vi "PJ1_GG.vi"() -> ()   [LabVIEW 2024]
uses:
  C:/Users/Windows 11/Downloads/Control 9.ctl
  <vilib>/Instr/_visa.llb/VISA Configure Serial Port (Instr).vi
  <vilib>/express/express analysis/Spectral/Block/exnSpectralBlock spectral measurements PSD poly.vi
  <vilib>/express/express analysis/Spectral/Block/exnSpectralBlock spectral measurements PSD DDT.vi
  <vilib>/express/express analysis/Spectral/XNode/ExpressSpectralMeasurementsBlockNode.xnode
panel:
  in  "Sample":i32
  in  "Rate":dbl
  out "EEG Str":string
  in  "Upper Cut-Off":dbl=40.0
  out "PSD":dynamicdata(graph)
  out "PSD MAX":dbl
  out "Index ที่มากที่สุด":i32
  out "max value":dbl
  out "B 18+1":dbl
  out "N 18+1":dbl
  in  "Aj 18+1":dbl
  out "B 18+1":dbl
  out "PSD 18+1":dbl
  out "B 18":dbl
  out "N 18":dbl
  in  "Aj 18":dbl
  out "B 18":dbl
  out "PSD 18":dbl
  out "B 18-1":dbl
  out "N 18-1":dbl
  in  "Aj 18-1":dbl
  out "B 18-1":dbl
  out "PSD 18-1":dbl
  out "9 Hz":dbl[](array[numeric])
  out "Max Index 9":i32
  out "PSD max 9":dbl
  out "PSD 9-1":dbl
  out "B 9-1":dbl
  in  "Aj 9-1":dbl
  out "N 9-1":dbl
  out "B 9-1":dbl
  out "PSD 9":dbl
  out "B 9":dbl
  in  "Aj 9":dbl
  out "N 9":dbl
  out "B 9":dbl
  out "PSD 9+1":dbl
  out "B 9+1":dbl
  in  "Aj 9+1":dbl
  out "N 9+1":dbl
  out "B 9+1":dbl
  out "8 Hz":dbl[](array[numeric])
  out "Max Index 8":i32
  out "PSD max 8":dbl
  out "B 16+1":dbl
  out "N 16+1":dbl
  in  "Aj  16+1":dbl
  out "B 16+1":dbl
  out "PSD  16+1":dbl
  out "B 16":dbl
  out "N  16":dbl
  in  "Aj  16":dbl
  out "B 16":dbl
  out "PSD  16":dbl
  out "B 16-1":dbl
  out "N  16-1":dbl
  in  "Aj   16-1":dbl
  out "B   16-1":dbl
  out "PSD 16-1":dbl
  out "B 8+1":dbl
  out "N 8+1":dbl
  in  "Aj  8+1":dbl
  out "B  8+1":dbl
  out "PSD 8+1":dbl
  out "B 8":dbl
  out "N  8":dbl
  in  "Aj  8":dbl
  out "B  8":dbl
  out "PSD 8":dbl
  out "B 8-1":dbl
  out "N  8-1":dbl
  in  "Aj  8-1":dbl
  out "B  8-1":dbl
  out "PSD 8-1":dbl
  out "PSD 14+1":dbl
  out "B 14+1":dbl
  in  "Aj 14+1":dbl
  out "N 14+1":dbl
  out "B 14+1":dbl
  out "PSD 14":dbl
  out "B 14":dbl
  in  "Aj 14":dbl
  out "N 14":dbl
  out "B 14":dbl
  out "PSD 14-1":dbl
  out "B 14-1":dbl
  in  "Aj 14-1":dbl
  out "N 14-1":dbl
  out "B 14-1":dbl
  out "PSD7+1":dbl
  out "B7+1":dbl
  in  "Aj7+1":dbl
  out "N7+1":dbl
  out "B7+1":dbl
  out "PSD 7":dbl
  out "B 7":dbl
  in  "Aj 7":dbl
  out "N7":dbl
  out "B7":dbl
  out "7 Hz":dbl[](array[numeric])
  out "Max Index 7":i32
  out "PSD max 7":dbl
  out "PSD 7-1":dbl
  out "B 7-1":dbl
  in  "Aj 7-1":dbl
  out "N7-1":dbl
  out "B7-1":dbl
  out "B12-1":dbl
  out "N12-1":dbl
  in  "Aj 12-1":dbl
  out "B 12-1":dbl
  out "PSD 12-1":dbl
  out "B12":dbl
  out "N12":dbl
  in  "Aj 12":dbl
  out "B12":dbl
  out "PSD 12":dbl
  out "B12+1":dbl
  out "N12+1":dbl
  in  "Aj 12+1":dbl
  out "B 12+1":dbl
  out "PSD 12+1":dbl
  out "B6+1":dbl
  out "N6+1":dbl
  in  "Aj 6+1":dbl
  out "B 6+1":dbl
  out "PSD 6+1":dbl
  out "B6":dbl
  out "N6":dbl
  in  "Aj 6":dbl
  out "B6":dbl
  out "PSD 6":dbl
  out "PSD 6-1":dbl
  out "6 Hz":dbl[](array[numeric])
  out "Max Index 6":i32
  out "PSD max 6":dbl
  out "B 6-1":dbl
  in  "Aj 6-1":dbl
  out "N6-1":dbl
  out "B6-1":dbl
  in  "Baseline":bool
  out "appended array":dbl[][](array[numeric])
  out "Filtered Signal":dynamicdata(graph)
  in  "Lower Cut-Off":dbl=1.0
  out "data":dbl[][](graph) caption="Raw Data"
  out "?":bool
  out "?":bool
  out "?":bool
  out "?":bool
  out "?":bool
  out "?":bool
  out "?":bool
  out "?":bool
  out "?":bool
  out "?":bool
  out "?":bool=TRUE
  out "?":bool=TRUE
  out "?":bool=TRUE
  out "?":bool=TRUE
  out "?":bool=TRUE
  out "?":bool=TRUE
  out "?":bool=TRUE
  out "?":bool=TRUE
  out "?":bool=TRUE
  out "?":bool=TRUE
  out "?":bool
  out "?":bool
  out "?":bool
  out "?":bool
  out "?":bool
  out "?":bool
  out "?":bool
  out "?":bool
  out "?":bool
  out "?":bool
  out "?":bool=TRUE
  out "?":bool=TRUE
  out "?":bool=TRUE
  out "?":bool=TRUE
  out "?":bool=TRUE
  out "?":bool=TRUE
  out "?":bool=TRUE
  out "?":bool=TRUE
  out "?":bool=TRUE
  out "?":bool=TRUE
  out "?":bool
  out "?":bool
  out "?":bool
  out "?":bool
  out "?":bool
  out "?":bool
  out "?":bool
  out "?":bool
  out "?":bool
  out "?":bool
  out "?":bool=TRUE
  out "?":bool=TRUE
  out "?":bool=TRUE
  out "?":bool=TRUE
  out "?":bool=TRUE
  out "?":bool=TRUE
  out "?":bool=TRUE
  out "?":bool=TRUE
  out "?":bool=TRUE
  out "?":bool=TRUE
  out "?":bool
  out "?":bool
  out "?":bool
  out "?":bool
  out "?":bool
  out "?":bool
  out "?":bool
  out "?":bool
  out "?":bool
  out "?":bool
  out "?":bool=TRUE
  out "?":bool=TRUE
  out "?":bool=TRUE
  out "?":bool=TRUE
  out "?":bool=TRUE
  out "?":bool=TRUE
  out "?":bool=TRUE
  out "?":bool=TRUE
  out "?":bool=TRUE
  out "?":bool=TRUE
  out "9 HZ":bool
  out "8 HZ":bool
  out "6 HZ":bool
  out "7 HZ":bool
  in  "Tab Control":enum32{"TAB 1", "TAB 2", "TAB 3", "TAB 4"}(tab)
  out "555":bool
  in  "MENU 4":bool
  in  "MENU 3":bool
  in  "MENU 2":bool
  in  "MENU":bool
  in  "start":bool
  in  "Text3":bool
  in  "Text2":bool
  in  "Backpage 2":T1
  out "String":string
  in  "Text1":bool
  in  "send":bool
  in  "Back":bool
  in  "1 3":bool
  in  "1 2":bool
  in  "1":bool
  out "String 2":string
  in  "SOS CALLING":bool
  in  "Blank Button 14":bool
  in  "LED":bool
  in  "Blank Button 12":bool
  in  "Back 4":bool
  in  "VISA resource name":refnum<visa-resource-name>
  # "Tel."
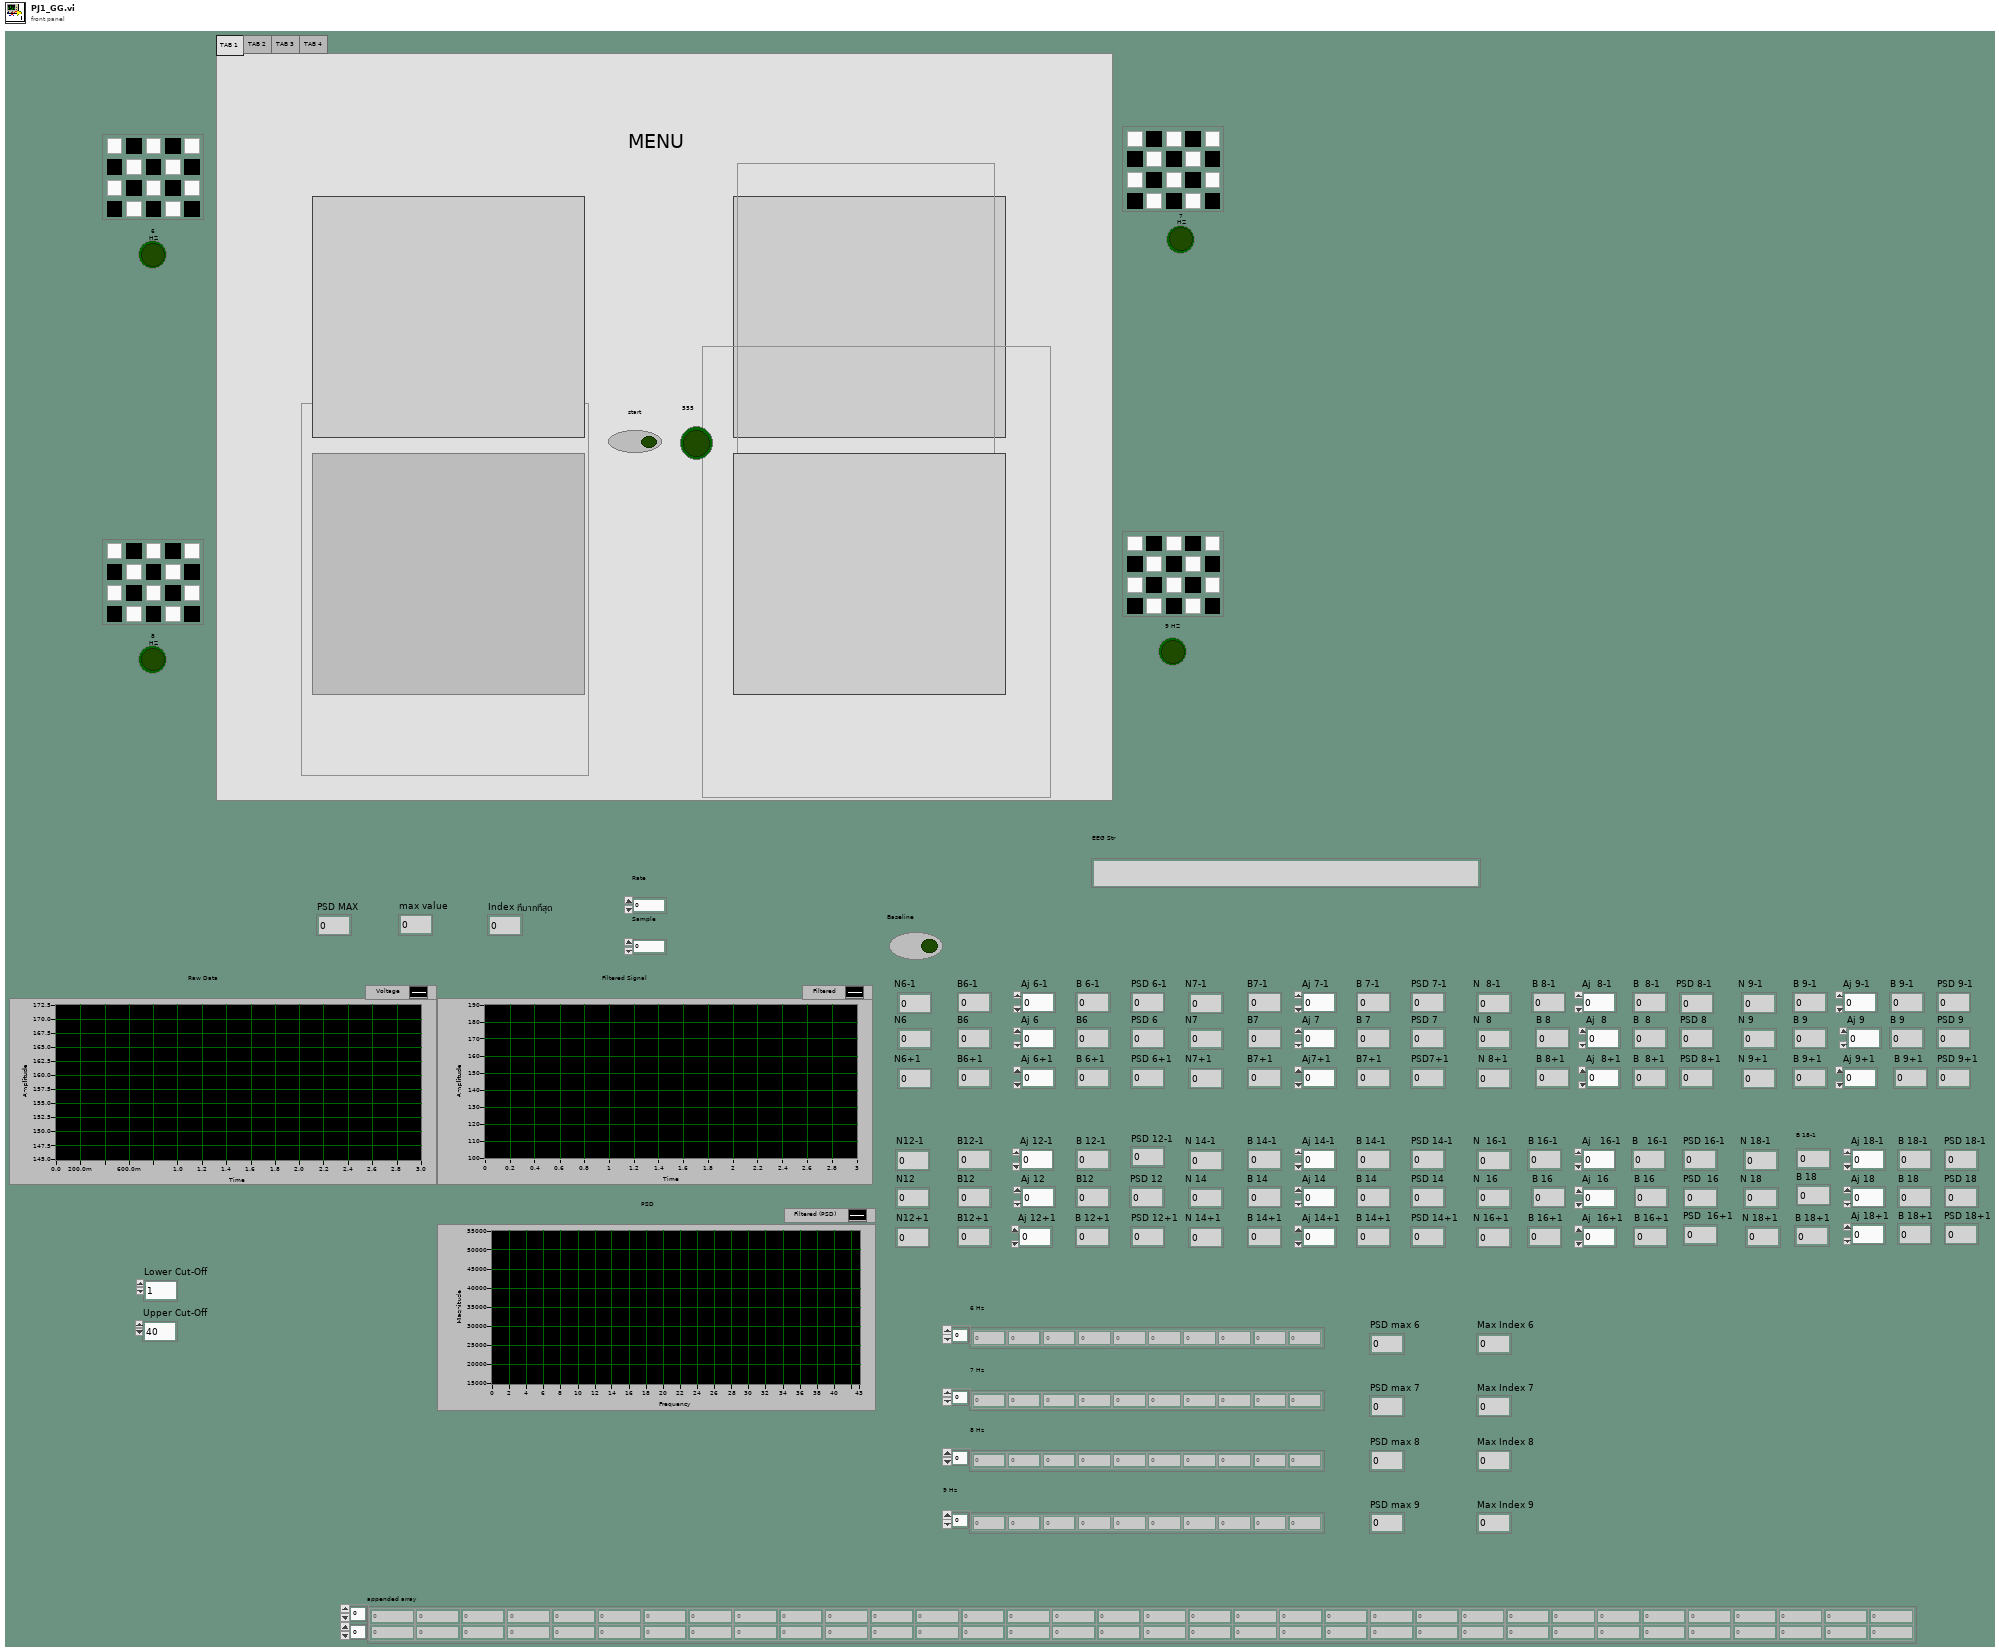
[diagram p1: front panel]
types:
  T1 = typedef "Control 9.ctl" = bool
  T2 = cluster{"averaging mode":u16, "weighting mode":u16, "number of averages":u32}
  T3 = cluster{"dB On (F)":bool, "unwrap phase (F)":bool, "convert to degree (F)":bool}
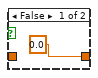
[diagram p3: hidden frame]
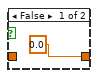
[diagram p5: hidden frame]
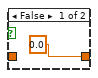
[diagram p7: hidden frame]
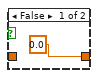
[diagram p9: hidden frame]
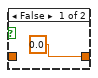
[diagram p11: hidden frame]
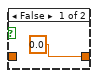
[diagram p13: hidden frame]
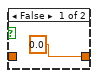
[diagram p15: hidden frame]
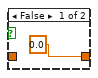
[diagram p17: hidden frame]
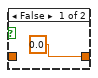
[diagram p19: hidden frame]
diagram:
  n1 = while {
    shift-right: [w16] -> _
    shift-left: "" -> [w18]
    stop <- FALSE stop-if-true
    n2 = event shown="[3] \"Back\": Value Change" {
      selector: _ -> [_ _ _ _]
      dyn-events: _ -> [_ _ _ _]
      timeout: _ -> [_ _ _ _]
      tunnel: w18 -> [_ _ _ _]
      tunnel: ["0622436287" "1669" " 0937529340" _] -> w16
      event "1 2": Value Change {
        n3 = event-data() -> ()  [unwired: 1 in, 6 out]
      }
      event "1": Value Change {
        n4 = event-data() -> ()  [unwired: 1 in, 6 out]
      }
      event "1 3": Value Change {
        n5 = event-data() -> ()  [unwired: 1 in, 6 out]
      }
      event "Back": Value Change {
        n6 = event-data() -> ()  [unwired: 1 in, 6 out]
        n7 = local write "Tab Control"(enum32{"TAB 1", "TAB 2", "TAB 3", "TAB 4"}."TAB 1" ("Tab Control")) -> ()
      }
    }
    "String 2" <- w16
  }
  n8 = String To IP(1:"127.0.0.1") -> (0:w5:u32)
  n9 = UDP Open(7:w5, 11:u16 5005 ("port")) -> (port=w4:refnum<k16>, 0:w3:errorcluster)  [unwired: 3 in, 1 out]
  n10 = while {
    stop <- FALSE stop-if-true
    n11 = while {
      tunnel: "start" -> [_]
      stop <- FALSE stop-if-true
      n12 = while {
        stop <- FALSE stop-if-true
        w63 = 83.3333
        # "6 HZ"
        n13 = for {
          N: 2 -> [_]
          tunnel: w63 -> [w67]
          i -> [w69]
          n14 = Wait (ms)(milliseconds to wait=w67) -> ()  [unwired: 1 out]
          n15 = Equal?(x=0, y=w69) -> (x = y?=→"?" →"?" →"?" →"?" →"?" →"?" →"?" →"?" →"?" →"?":bool)
        }
        n16 = for {
          N: 2 -> [_]
          tunnel: w63 -> [w71]
          i -> [w72]
          n17 = Wait (ms)(milliseconds to wait=w71) -> ()  [unwired: 1 out]
          n18 = Equal?(x=1, y=w72) -> (x = y?=→"?" →"?" →"?" →"?" →"?" →"?" →"?" →"?" →"?" →"?":bool)
        }
      }
      n19 = while {
        stop <- FALSE stop-if-true
        w51 = 71.428571
        # "7 HZ"
        n20 = for {
          N: 2 -> [_]
          tunnel: w51 -> [w55]
          i -> [w57]
          n21 = Wait (ms)(milliseconds to wait=w55) -> ()  [unwired: 1 out]
          n22 = Equal?(x=0, y=w57) -> (x = y?=→"?" →"?" →"?" →"?" →"?" →"?" →"?" →"?" →"?" →"?":bool)
        }
        n23 = for {
          N: 2 -> [_]
          tunnel: w51 -> [w59]
          i -> [w60]
          n24 = Wait (ms)(milliseconds to wait=w59) -> ()  [unwired: 1 out]
          n25 = Equal?(x=1, y=w60) -> (x = y?=→"?" →"?" →"?" →"?" →"?" →"?" →"?" →"?" →"?" →"?":bool)
        }
      }
      n26 = while {
        stop <- FALSE stop-if-true
        w39 = 62.5
        # "8 HZ"
        n27 = for {
          N: 2 -> [_]
          tunnel: w39 -> [w43]
          i -> [w45]
          n28 = Wait (ms)(milliseconds to wait=w43) -> ()  [unwired: 1 out]
          n29 = Equal?(x=0, y=w45) -> (x = y?=→"?" →"?" →"?" →"?" →"?" →"?" →"?" →"?" →"?" →"?":bool)
        }
        n30 = for {
          N: 2 -> [_]
          tunnel: w39 -> [w47]
          i -> [w48]
          n31 = Wait (ms)(milliseconds to wait=w47) -> ()  [unwired: 1 out]
          n32 = Equal?(x=1, y=w48) -> (x = y?=→"?" →"?" →"?" →"?" →"?" →"?" →"?" →"?" →"?" →"?":bool)
        }
      }
      n33 = while {
        stop <- FALSE stop-if-true
        w27 = 55.5555
        # "9 HZ"
        n34 = for {
          N: 2 -> [_]
          tunnel: w27 -> [w31]
          i -> [w33]
          n35 = Wait (ms)(milliseconds to wait=w31) -> ()  [unwired: 1 out]
          n36 = Equal?(x=0, y=w33) -> (x = y?=→"?" →"?" →"?" →"?" →"?" →"?" →"?" →"?" →"?" →"?":bool)
        }
        n37 = for {
          N: 2 -> [_]
          tunnel: w27 -> [w35]
          i -> [w36]
          n38 = Wait (ms)(milliseconds to wait=w35) -> ()  [unwired: 1 out]
          n39 = Equal?(x=1, y=w36) -> (x = y?=→"?" →"?" →"?" →"?" →"?" →"?" →"?" →"?" →"?" →"?":bool)
        }
      }
    }
  }
  n40 = while {
    tunnel: w4 -> [w88]
    tunnel: w3 -> [w87]
    tunnel: [w85] -> w2
    tunnel: [w84] -> w1
    stop <- FALSE stop-if-true
    n41 = UDP Read(connection ID=w88, timeout ms (25000)=500, 8:w87) -> (data out=w79:string, error out=w85:errorcluster, 3:w84:refnum<k16>)  [unwired: 1 in, 2 out]
    "EEG Str" <- w79
    n42 = Spreadsheet String To Array(delimiter (Tab)=",", format string="%f", spreadsheet string=w79, array type (2D Dbl)=0.0) -> (array=→"data":dbl[][])
    n43 = Bundle By Name("dt"=0.005) -> (w74:waveform(dbl))  [unwired: 3 in]
    n44 = call "Convert to Dynamic Data"("2D Array"=w74) -> ("Dynamic Data Type"=w81:dynamicdata)  [unwired: 3 in]
    n45 = Divide(x="Rate", y="Sample") -> (x/y=w178:dbl)
    n46 = call "Filter"("Lower Cut-Off"="Lower Cut-Off", "Upper Cut-Off"="Upper Cut-Off", "Signal"=w81) -> ("Filtered Signal"=w467:dynamicdata)  [unwired: 7 in, 1 out]
    "Filtered Signal" <- w467
    n47 = Divide(x=8.0, y=w178) -> (x/y=w278:dbl)
    n48 = Divide(x=16.0, y=w178) -> (x/y=w230:dbl)
    n49 = Divide(x=14.0, y=w178) -> (x/y=w303:dbl)
    n50 = Divide(x=18.0, y=w178) -> (x/y=w153:dbl)
    n51 = xnode "Spectral Measurements"("Signals"=w467) -> ("PSD"=w115:dynamicdata)  [unwired: 1 in, 1 out]
    "PSD" <- w115
    n52 = Divide(x=9.0, y=w178) -> (x/y=w196:dbl)
    n53 = Divide(x=7.0, y=w178) -> (x/y=w320:dbl)
    n54 = Divide(x=12.0, y=w178) -> (x/y=w389:dbl)
    n55 = Divide(x=6.0, y=w178) -> (x/y=w438:dbl)
    n56 = call "Convert from Dynamic Data"("Dynamic Data Type"=w115) -> ("Array"=w466:dbl[])  [unwired: 3 in]
    n57 = Decrement(x=w196) -> (x-1=w227:dbl)
    n58 = Increment(x=w196) -> (x+1=w195:dbl)
    n59 = Increment(x=w153) -> (x+1=w142:dbl)
    n60 = Decrement(x=w153) -> (x-1=w167:dbl)
    n61 = Decrement(x=w303) -> (x-1=w332:dbl)
    n62 = Increment(x=w278) -> (x+1=w268:dbl)
    n63 = Decrement(x=w230) -> (x-1=w253:dbl)
    n64 = Decrement(x=w438) -> (x-1=w451:dbl)
    n65 = Decrement(x=w320) -> (x-1=w361:dbl)
    "PSD 7-1" <- w361
    n66 = Increment(x=w320) -> (x+1=w346:dbl)
    n67 = Decrement(x=w278) -> (x-1=w291:dbl)
    n68 = Increment(x=w230) -> (x+1=w229:dbl)
    n69 = Increment(x=w438) -> (x+1=w427:dbl)
    n70 = Increment(x=w303) -> (x+1=w309:dbl)
    n71 = Decrement(x=w389) -> (x-1=w394:dbl)
    n72 = Increment(x=w389) -> (x+1=w388:dbl)
    n73 = Build Array(w466) -> (w143:dbl[][])
    "appended array" <- w143
    n74 = Index Array(array=w143, index (row)=0, index (col)=w253) -> (element=w264:dbl)
    "PSD 16-1" <- w264
    n75 = Index Array(array=w143, index (row)=0 ("disabled index (row)"), index (col)=w229) -> (element=w241:dbl)
    "PSD  16+1" <- w241
    n76 = Index Array(array=w143, index (row)=0 ("disabled index (row)"), index (col)=w230) -> (element=w243:dbl)
    "PSD  16" <- w243
    n77 = Index Array(array=w143, index (row)=0, index (col)=w309) -> (element=w310:dbl)
    "PSD 14+1" <- w310
    n78 = Index Array(array=w143, index (row)=0 ("disabled index (row)"), index (col)=w167) -> (element=w165:dbl)
    "PSD 18-1" <- w165
    n79 = Index Array(array=w143, index (row)=0, index (col)=w268) -> (element=w266:dbl)
    "PSD 8+1" <- w266
    n80 = Index Array(array=w143, index (row)=0 ("disabled index (row)"), index (col)=w142) -> (element=w139:dbl)
    "PSD 18+1" <- w139
    n81 = Index Array(array=w143, index (row)=0, index (col)=w195) -> (element=w184:dbl)
    "PSD 9-1" <- w184
    n82 = Index Array(array=w143, index (row)=0, index (col)=w278) -> (element=w289:dbl)
    "PSD 8" <- w289
    n83 = Index Array(array=w143, index (row)=0 ("disabled index (row)"), index (col)=w153) -> (element=w154:dbl)
    "PSD 18" <- w154
    n84 = Index Array(array=w143, index (row)=0, index (col)=w291) -> (element=w290:dbl)
    "PSD 8-1" <- w290
    n85 = Index Array(array=w143, index (row)=0, index (col)=w196) -> (element=w197:dbl)
    "PSD 9" <- w197
    n86 = Index Array(array=w143, index (row)=0, index (col)=w227) -> (element=w208:dbl)
    "PSD 9+1" <- w208
    n87 = Index Array(array=w143, index (row)=0, index (col)=w332) -> (element=w334:dbl)
    "PSD 14-1" <- w334
    n88 = Index Array(array=w143, index (row)=0, index (col)=w303) -> (element=w321:dbl)
    "PSD 14" <- w321
    n89 = Index Array(array=w143, index (row)=0, index (col)=w361) -> ()  [unwired: 1 out]
    n90 = Index Array(array=w143, index (row)=0 ("disabled index (row)"), index (col)=w320) -> (element=w358:dbl)
    "PSD 7" <- w358
    n91 = Index Array(array=w143, index (row)=0, index (col)=w346) -> (element=w347:dbl)
    "PSD7+1" <- w347
    n92 = Index Array(array=w143, index (row)=0 ("disabled index (row)"), index (col)=w427) -> (element=w425:dbl)
    "PSD 6+1" <- w425
    n93 = Index Array(array=w143, index (row)=0, index (col)=w394) -> (element=w393:dbl)
    "PSD 12-1" <- w393
    n94 = Index Array(array=w143, index (row)=0 ("disabled index (row)"), index (col)=w389) -> (element=w390:dbl)
    "PSD 12" <- w390
    n95 = Index Array(array=w143, index (row)=0 ("disabled index (row)"), index (col)=w388) -> (element=w386:dbl)
    "PSD 12+1" <- w386
    n96 = Index Array(array=w143, index (row)=0, index (col)=w438) -> (element=w439:dbl)
    "PSD 6" <- w439
    n97 = Index Array(array=w143, index (row)=0, index (col)=w451) -> (element=w458:dbl)
    "PSD 6-1" <- w458
    n98 = feedback #1() -> (w91:dbl)  [unwired: 1 in]
    "B 18" <- w91
    n99 = case shown="False" "Baseline" {
      tunnel: w154 -> [_ w478]
      tunnel: [w477 w478] -> w156
      tunnel: w91 -> [w477 _]
      frame False {
      }
      frame True {
      }
    }
    n100 = feedback-in #1(w156) -> ()
    n101 = feedback #2() -> (w92:dbl)  [unwired: 1 in]
    "B 18-1" <- w92
    n102 = case shown="False" "Baseline" {
      tunnel: w165 -> [_ w482]
      tunnel: [w481 w482] -> w176
      tunnel: w92 -> [w481 _]
      frame False {
      }
      frame True {
      }
    }
    n103 = feedback-in #2(w176) -> ()
    n104 = feedback #3() -> (w90:dbl)  [unwired: 1 in]
    "B 18+1" <- w90
    n105 = case shown="False" "Baseline" {
      tunnel: w139 -> [_ w474]
      tunnel: [w473 w474] -> w152
      tunnel: w90 -> [w473 _]
      frame False {
      }
      frame True {
      }
    }
    n106 = feedback-in #3(w152) -> ()
    n107 = feedback #4() -> (w98:dbl)  [unwired: 1 in]
    "B 16-1" <- w98
    n108 = case shown="True" "Baseline" {
      tunnel: w264 -> [_ w506]
      tunnel: [w505 w506] -> w254
      tunnel: w98 -> [w505 _]
      frame False {
      }
      frame True {
      }
    }
    n109 = feedback-in #4(w254) -> ()
    n110 = feedback #5() -> (w96:dbl)  [unwired: 1 in]
    "B 16+1" <- w96
    n111 = case shown="True" "Baseline" {
      tunnel: w241 -> [_ w498]
      tunnel: [w497 w498] -> w232
      tunnel: w96 -> [w497 _]
      frame False {
      }
      frame True {
      }
    }
    n112 = feedback-in #5(w232) -> ()
    n113 = feedback #6() -> (w97:dbl)  [unwired: 1 in]
    "B 16" <- w97
    n114 = case shown="True" "Baseline" {
      tunnel: w243 -> [_ w502]
      tunnel: [w501 w502] -> w252
      tunnel: w97 -> [w501 _]
      frame False {
      }
      frame True {
      }
    }
    n115 = feedback-in #6(w252) -> ()
    n116 = feedback #7() -> (w99:dbl)  [unwired: 1 in]
    "B 8+1" <- w99
    n117 = case shown="True" "Baseline" {
      tunnel: w266 -> [_ w510]
      tunnel: [w509 w510] -> w277
      tunnel: w99 -> [w509 _]
      frame False {
      }
      frame True {
      }
    }
    n118 = feedback-in #7(w277) -> ()
    n119 = feedback #8() -> (w102:dbl)  [unwired: 1 in]
    "B 14+1" <- w102
    n120 = case shown="True" "Baseline" {
      tunnel: w310 -> [_ w522]
      tunnel: [w521 w522] -> w311
      tunnel: w102 -> [w521 _]
      frame False {
      }
      frame True {
      }
    }
    n121 = feedback-in #8(w311) -> ()
    n122 = feedback #9() -> (w100:dbl)  [unwired: 1 in]
    "B 8" <- w100
    n123 = case shown="True" "Baseline" {
      tunnel: w289 -> [_ w514]
      tunnel: [w513 w514] -> w280
      tunnel: w100 -> [w513 _]
      frame False {
      }
      frame True {
      }
    }
    n124 = feedback-in #9(w280) -> ()
    n125 = feedback #10() -> (w94:dbl)  [unwired: 1 in]
    "B 9" <- w94
    n126 = case shown="False" "Baseline" {
      tunnel: w197 -> [_ w490]
      tunnel: [w489 w490] -> w198
      tunnel: w94 -> [w489 _]
      frame False {
      }
      frame True {
      }
    }
    n127 = feedback-in #10(w198) -> ()
    n128 = feedback #11() -> (w101:dbl)  [unwired: 1 in]
    "B 8-1" <- w101
    n129 = case shown="True" "Baseline" {
      tunnel: w290 -> [_ w518]
      tunnel: [w517 w518] -> w301
      tunnel: w101 -> [w517 _]
      frame False {
      }
      frame True {
      }
    }
    n130 = feedback-in #11(w301) -> ()
    n131 = feedback #12() -> (w95:dbl)  [unwired: 1 in]
    "B 9+1" <- w95
    n132 = case shown="True" "Baseline" {
      tunnel: w208 -> [_ w494]
      tunnel: [w493 w494] -> w209
      tunnel: w95 -> [w493 _]
      frame False {
      }
      frame True {
      }
    }
    n133 = feedback-in #12(w209) -> ()
    n134 = feedback #13() -> (w110:dbl)  [unwired: 1 in]
    "B12-1" <- w110
    n135 = case shown="True" "Baseline" {
      tunnel: w393 -> [_ w554]
      tunnel: [w553 w554] -> w405
      tunnel: w110 -> [w553 _]
      frame False {
      }
      frame True {
      }
    }
    n136 = feedback-in #13(w405) -> ()
    n137 = feedback #14() -> (w104:dbl)  [unwired: 1 in]
    "B 14-1" <- w104
    n138 = case shown="True" "Baseline" {
      tunnel: w334 -> [_ w530]
      tunnel: [w529 w530] -> w335
      tunnel: w104 -> [w529 _]
      frame False {
      }
      frame True {
      }
    }
    n139 = feedback-in #14(w335) -> ()
    n140 = feedback #15() -> (w93:dbl)  [unwired: 1 in]
    "B 9-1" <- w93
    n141 = case shown="False" "Baseline" {
      tunnel: w184 -> [_ w486]
      tunnel: [w485 w486] -> w185
      tunnel: w93 -> [w485 _]
      frame False {
      }
      frame True {
      }
    }
    n142 = feedback-in #15(w185) -> ()
    n143 = feedback #16() -> (w111:dbl)  [unwired: 1 in]
    "B6+1" <- w111
    n144 = case shown="True" "Baseline" {
      tunnel: w425 -> [_ w558]
      tunnel: [w557 w558] -> w428
      tunnel: w111 -> [w557 _]
      frame False {
      }
      frame True {
      }
    }
    n145 = feedback-in #16(w428) -> ()
    n146 = feedback #17() -> (w112:dbl)  [unwired: 1 in]
    "B6" <- w112
    n147 = case shown="True" "Baseline" {
      tunnel: w439 -> [_ w562]
      tunnel: [w561 w562] -> w449
      tunnel: w112 -> [w561 _]
      frame False {
      }
      frame True {
      }
    }
    n148 = feedback-in #17(w449) -> ()
    n149 = feedback #18() -> (w113:dbl)  [unwired: 1 in]
    "B6-1" <- w113
    n150 = case shown="True" "Baseline" {
      tunnel: w458 -> [_ w566]
      tunnel: [w565 w566] -> w450
      tunnel: w113 -> [w565 _]
      frame False {
      }
      frame True {
      }
    }
    n151 = feedback-in #18(w450) -> ()
    n152 = feedback #19() -> (w103:dbl)  [unwired: 1 in]
    "B 14" <- w103
    n153 = case shown="True" "Baseline" {
      tunnel: w321 -> [_ w526]
      tunnel: [w525 w526] -> w323
      tunnel: w103 -> [w525 _]
      frame False {
      }
      frame True {
      }
    }
    n154 = feedback-in #19(w323) -> ()
    n155 = feedback #20() -> (w108:dbl)  [unwired: 1 in]
    "B12+1" <- w108
    n156 = case shown="True" "Baseline" {
      tunnel: w386 -> [_ w546]
      tunnel: [w545 w546] -> w423
      tunnel: w108 -> [w545 _]
      frame False {
      }
      frame True {
      }
    }
    n157 = feedback-in #20(w423) -> ()
    n158 = Add(x=w91, y="Aj 18") -> (x+y=w160:dbl)
    "B 18" <- w160
    n159 = Add(x=w92, y="Aj 18-1") -> (x+y=w172:dbl)
    "B 18-1" <- w172
    n160 = Add(x=w90, y="Aj 18+1") -> (x+y=w148:dbl)
    "B 18+1" <- w148
    n161 = feedback #21() -> (w109:dbl)  [unwired: 1 in]
    "B12" <- w109
    n162 = case shown="True" "Baseline" {
      tunnel: w390 -> [_ w550]
      tunnel: [w549 w550] -> w406
      tunnel: w109 -> [w549 _]
      frame False {
      }
      frame True {
      }
    }
    n163 = feedback-in #21(w406) -> ()
    n164 = Add(x=w98, y="Aj   16-1") -> (x+y=w258:dbl)
    "B   16-1" <- w258
    n165 = Add(x=w96, y="Aj  16+1") -> (x+y=w236:dbl)
    "B 16+1" <- w236
    n166 = Add(x=w97, y="Aj  16") -> (x+y=w248:dbl)
    "B 16" <- w248
    n167 = Add(x=w99, y="Aj  8+1") -> (x+y=w273:dbl)
    "B  8+1" <- w273
    n168 = Add(x=w102, y="Aj 14+1") -> (x+y=w315:dbl)
    "B 14+1" <- w315
    n169 = Add(x=w100, y="Aj  8") -> (x+y=w284:dbl)
    "B  8" <- w284
    n170 = Add(x=w94, y="Aj 9") -> (x+y=w202:dbl)
    "B 9" <- w202
    n171 = Add(x=w101, y="Aj  8-1") -> (x+y=w297:dbl)
    "B  8-1" <- w297
    n172 = Add(x=w95, y="Aj 9+1") -> (x+y=w213:dbl)
    "B 9+1" <- w213
    n173 = Add(x=w110, y="Aj 12-1") -> (x+y=w401:dbl)
    "B 12-1" <- w401
    n174 = Add(x=w104, y="Aj 14-1") -> (x+y=w339:dbl)
    "B 14-1" <- w339
    n175 = Add(x=w93, y="Aj 9-1") -> (x+y=w189:dbl)
    "B 9-1" <- w189
    n176 = Multiply(x=w91, y=5.0) -> (x*y=w163:dbl)
    "N 18" <- w163
    n177 = Add(x=w111, y="Aj 6+1") -> (x+y=w432:dbl)
    "B 6+1" <- w432
    n178 = Multiply(x=w92, y=5.0) -> (x*y=w169:dbl)
    "N 18-1" <- w169
    n179 = Multiply(x=w90, y=5.0) -> (x*y=w145:dbl)
    "N 18+1" <- w145
    n180 = feedback #22() -> (w105:dbl)  [unwired: 1 in]
    "B7+1" <- w105
    n181 = case shown="True" "Baseline" {
      tunnel: w347 -> [_ w534]
      tunnel: [w533 w534] -> w349
      tunnel: w105 -> [w533 _]
      frame False {
      }
      frame True {
      }
    }
    n182 = feedback-in #22(w349) -> ()
    n183 = feedback #23() -> (w106:dbl)  [unwired: 1 in]
    "B7" <- w106
    n184 = case shown="True" "Baseline" {
      tunnel: w358 -> [_ w538]
      tunnel: [w537 w538] -> w362
      tunnel: w106 -> [w537 _]
      frame False {
      }
      frame True {
      }
    }
    n185 = feedback-in #23(w362) -> ()
    n186 = Multiply(x=w98, y=5.0) -> (x*y=w261:dbl)
    "N  16-1" <- w261
    n187 = Multiply(x=w96, y=5.0) -> (x*y=w239:dbl)
    "N 16+1" <- w239
    n188 = Multiply(x=w97, y=5.0) -> (x*y=w245:dbl)
    "N  16" <- w245
    n189 = Multiply(x=w99, y=5.0) -> (x*y=w270:dbl)
    "N 8+1" <- w270
    n190 = feedback #24() -> (w107:dbl)  [unwired: 1 in]
    "B7-1" <- w107
    n191 = case shown="False" "Baseline" {
      tunnel: w361 -> [_ w542]
      tunnel: [w541 w542] -> w375
      tunnel: w107 -> [w541 _]
      frame False {
      }
      frame True {
      }
    }
    n192 = feedback-in #24(w375) -> ()
    n193 = Add(x=w112, y="Aj 6") -> (x+y=w445:dbl)
    "B6" <- w445
    n194 = Add(x=w113, y="Aj 6-1") -> (x+y=w459:dbl)
    "B 6-1" <- w459
    n195 = Add(x=w103, y="Aj 14") -> (x+y=w327:dbl)
    "B 14" <- w327
    n196 = Multiply(x=w102, y=5.0) -> (x*y=w318:dbl)
    "N 14+1" <- w318
    n197 = Multiply(x=w100, y=5.0) -> (x*y=w287:dbl)
    "N  8" <- w287
    n198 = Multiply(x=w94, y=5.0) -> (x*y=w205:dbl)
    "N 9" <- w205
    n199 = Multiply(x=w101, y=5.0) -> (x*y=w294:dbl)
    "N  8-1" <- w294
    n200 = Multiply(x=w95, y=5.0) -> (x*y=w216:dbl)
    "N 9+1" <- w216
    n201 = Add(x=w108, y="Aj 12+1") -> (x+y=w419:dbl)
    "B 12+1" <- w419
    n202 = Multiply(x=w110, y=5.0) -> (x*y=w398:dbl)
    "N12-1" <- w398
    n203 = Multiply(x=w104, y=5.0) -> (x*y=w342:dbl)
    "N 14-1" <- w342
    n204 = Add(x=w109, y="Aj 12") -> (x+y=w410:dbl)
    "B12" <- w410
    n205 = Multiply(x=w93, y=5.0) -> (x*y=w192:dbl)
    "N 9-1" <- w192
    n206 = Multiply(x=w111, y=5.0) -> (x*y=w435:dbl)
    "N6+1" <- w435
    n207 = Greater?(x=w154, y=w160) -> (0:w161:bool)
    n208 = Greater?(x=w165, y=w172) -> (0:w171:bool)
    n209 = Greater?(x=w139, y=w148) -> (0:w147:bool)
    n210 = Less?(x=w154, y=w163) -> (x < y?=w162:bool)
    n211 = Less?(x=w165, y=w169) -> (x < y?=w170:bool)
    n212 = Multiply(x=w112, y=5.0) -> (x*y=w442:dbl)
    "N6" <- w442
    n213 = Multiply(x=w113, y=5.0) -> (x*y=w462:dbl)
    "N6-1" <- w462
    n214 = Multiply(x=w103, y=5.0) -> (x*y=w330:dbl)
    "N 14" <- w330
    n215 = Greater?(x=w264, y=w258) -> (0:w259:bool)
    n216 = Less?(x=w139, y=w145) -> (x < y?=w146:bool)
    n217 = Greater?(x=w241, y=w236) -> (0:w237:bool)
    n218 = Greater?(x=w243, y=w248) -> (0:w247:bool)
    n219 = Greater?(x=w266, y=w273) -> (0:w272:bool)
    n220 = Less?(x=w264, y=w261) -> (x < y?=w260:bool)
    n221 = Less?(x=w241, y=w239) -> (x < y?=w238:bool)
    n222 = Multiply(x=w108, y=5.0) -> (x*y=w416:dbl)
    "N12+1" <- w416
    n223 = Less?(x=w243, y=w245) -> (x < y?=w246:bool)
    n224 = Greater?(x=w310, y=w315) -> (0:w316:bool)
    n225 = Less?(x=w266, y=w270) -> (x < y?=w271:bool)
    n226 = Greater?(x=w289, y=w284) -> (0:w285:bool)
    n227 = Greater?(x=w197, y=w202) -> (0:w203:bool)
    n228 = Multiply(x=w109, y=5.0) -> (x*y=w413:dbl)
    "N12" <- w413
    n229 = Add(x=w105, y="Aj7+1") -> (x+y=w353:dbl)
    "B7+1" <- w353
    n230 = Less?(x=w310, y=w318) -> (x < y?=w317:bool)
    n231 = Greater?(x=w290, y=w297) -> (0:w296:bool)
    n232 = Less?(x=w289, y=w287) -> (x < y?=w286:bool)
    n233 = Less?(x=w197, y=w205) -> (x < y?=w204:bool)
    n234 = Greater?(x=w208, y=w213) -> (0:w214:bool)
    n235 = Add(x=w106, y="Aj 7") -> (x+y=w366:dbl)
    "B 7" <- w366
    n236 = Less?(x=w290, y=w294) -> (x < y?=w295:bool)
    n237 = Greater?(x=w393, y=w401) -> (0:w400:bool)
    n238 = Greater?(x=w334, y=w339) -> (0:w340:bool)
    n239 = Less?(x=w208, y=w216) -> (x < y?=w215:bool)
    n240 = Greater?(x=w184, y=w189) -> (0:w190:bool)
    n241 = Add(x=w107, y="Aj 7-1") -> (x+y=w379:dbl)
    "B 7-1" <- w379
    n242 = Greater?(x=w425, y=w432) -> (0:w433:bool)
    n243 = Less?(x=w393, y=w398) -> (x < y?=w399:bool)
    n244 = Less?(x=w334, y=w342) -> (x < y?=w341:bool)
    n245 = Less?(x=w184, y=w192) -> (x < y?=w191:bool)
    n246 = Less?(x=w425, y=w435) -> (x < y?=w434:bool)
    n247 = And(x=w162, y=w161) -> (x .and. y?=w159:bool)
    n248 = Subtract(x=w154, y=w160) -> (x-y=w158:dbl)
    n249 = And(x=w170, y=w171) -> (x .and. y?=w173:bool)
    n250 = Greater?(x=w439, y=w445) -> (0:w444:bool)
    n251 = Subtract(x=w165, y=w172) -> (x-y=w174:dbl)
    n252 = Greater?(x=w458, y=w459) -> (0:w460:bool)
    n253 = Greater?(x=w321, y=w327) -> (0:w328:bool)
    n254 = And(x=w146, y=w147) -> (x .and. y?=w149:bool)
    n255 = Subtract(x=w139, y=w148) -> (x-y=w150:dbl)
    n256 = Less?(x=w439, y=w442) -> (x < y?=w443:bool)
    n257 = Less?(x=w458, y=w462) -> (x < y?=w461:bool)
    n258 = Less?(x=w321, y=w330) -> (x < y?=w329:bool)
    n259 = And(x=w260, y=w259) -> (x .and. y?=w257:bool)
    n260 = Multiply(x=w105, y=5.0) -> (x*y=w356:dbl)
    "N7+1" <- w356
    n261 = Subtract(x=w264, y=w258) -> (x-y=w256:dbl)
    n262 = And(x=w238, y=w237) -> (x .and. y?=w235:bool)
    n263 = Subtract(x=w241, y=w236) -> (x-y=w234:dbl)
    n264 = Greater?(x=w386, y=w419) -> (0:w418:bool)
    n265 = Multiply(x=w106, y=5.0) -> (x*y=w369:dbl)
    "N7" <- w369
    n266 = And(x=w246, y=w247) -> (x .and. y?=w249:bool)
    n267 = And(x=w271, y=w272) -> (x .and. y?=w274:bool)
    n268 = Subtract(x=w243, y=w248) -> (x-y=w250:dbl)
    n269 = Subtract(x=w266, y=w273) -> (x-y=w275:dbl)
    n270 = Greater?(x=w390, y=w410) -> (0:w411:bool)
    n271 = Less?(x=w386, y=w416) -> (x < y?=w417:bool)
    n272 = And(x=w317, y=w316) -> (x .and. y?=w314:bool)
    n273 = Subtract(x=w310, y=w315) -> (x-y=w313:dbl)
    n274 = Multiply(x=w107, y=5.0) -> (x*y=w382:dbl)
    "N7-1" <- w382
    n275 = And(x=w286, y=w285) -> (x .and. y?=w283:bool)
    n276 = Subtract(x=w289, y=w284) -> (x-y=w282:dbl)
    n277 = And(x=w204, y=w203) -> (x .and. y?=w201:bool)
    n278 = Subtract(x=w197, y=w202) -> (x-y=w200:dbl)
    n279 = Less?(x=w390, y=w413) -> (x < y?=w412:bool)
    n280 = And(x=w295, y=w296) -> (x .and. y?=w298:bool)
    n281 = Subtract(x=w290, y=w297) -> (x-y=w299:dbl)
    n282 = And(x=w215, y=w214) -> (x .and. y?=w212:bool)
    n283 = Subtract(x=w208, y=w213) -> (x-y=w211:dbl)
    n284 = And(x=w399, y=w400) -> (x .and. y?=w402:bool)
    n285 = Subtract(x=w393, y=w401) -> (x-y=w403:dbl)
    n286 = And(x=w341, y=w340) -> (x .and. y?=w338:bool)
    n287 = Subtract(x=w334, y=w339) -> (x-y=w337:dbl)
    n288 = And(x=w191, y=w190) -> (x .and. y?=w188:bool)
    n289 = Subtract(x=w184, y=w189) -> (x-y=w187:dbl)
    n290 = Subtract(x=w425, y=w432) -> (x-y=w430:dbl)
    n291 = And(x=w434, y=w433) -> (x .and. y?=w431:bool)
    n292 = And(x=w461, y=w460) -> (x .and. y?=w457:bool)
    n293 = Subtract(x=w439, y=w445) -> (x-y=w447:dbl)
    n294 = And(x=w329, y=w328) -> (x .and. y?=w326:bool)
    n295 = Subtract(x=w458, y=w459) -> (x-y=w456:dbl)
    n296 = Greater?(x=w347, y=w353) -> (0:w354:bool)
    n297 = Subtract(x=w321, y=w327) -> (x-y=w325:dbl)
    n298 = Greater?(x=w358, y=w366) -> (0:w367:bool)
    n299 = And(x=w443, y=w444) -> (x .and. y?=w446:bool)
    n300 = Less?(x=w347, y=w356) -> (x < y?=w355:bool)
    n301 = Less?(x=w358, y=w369) -> (x < y?=w368:bool)
    n302 = Subtract(x=w386, y=w419) -> (x-y=w421:dbl)
    n303 = Greater?(x=w361, y=w379) -> (0:w380:bool)
    n304 = Subtract(x=w390, y=w410) -> (x-y=w408:dbl)
    n305 = And(x=w417, y=w418) -> (x .and. y?=w420:bool)
    n306 = Less?(x=w361, y=w382) -> (x < y?=w381:bool)
    n307 = And(x=w412, y=w411) -> (x .and. y?=w409:bool)
    n308 = And(x=w355, y=w354) -> (x .and. y?=w352:bool)
    n309 = Subtract(x=w347, y=w353) -> (x-y=w351:dbl)
    n310 = And(x=w368, y=w367) -> (x .and. y?=w365:bool)
    n311 = Subtract(x=w358, y=w366) -> (x-y=w364:dbl)
    n312 = And(x=w381, y=w380) -> (x .and. y?=w378:bool)
    n313 = Subtract(x=w361, y=w379) -> (x-y=w377:dbl)
    n314 = case shown="True" w402 {
      tunnel: w403 -> [_ w552]
      tunnel: [0.0 w552] -> w392
      frame False {
      }
      frame True {
      }
    }
    n315 = case shown="True" w431 {
      tunnel: w430 -> [_ w556]
      tunnel: [0.0 w556] -> w424
      frame False {
      }
      frame True {
      }
    }
    n316 = case shown="False" w457 {
      tunnel: w456 -> [_ w564]
      tunnel: [0.0 w564] -> w454
      frame False {
      }
      frame True {
      }
    }
    n317 = case shown="False" w446 {
      tunnel: w447 -> [_ w560]
      tunnel: [0.0 w560] -> w437
      frame False {
      }
      frame True {
      }
    }
    n318 = case shown="True" w420 {
      tunnel: w421 -> [_ w544]
      tunnel: [0.0 w544] -> w384
      frame False {
      }
      frame True {
      }
    }
    n319 = case shown="True" w159 {
      tunnel: w158 -> [_ w476]
      tunnel: [0.0 w476] -> w137
      frame False {
      }
      frame True {
      }
    }
    n320 = case shown="True" w409 {
      tunnel: w408 -> [_ w548]
      tunnel: [0.0 w548] -> w385
      frame False {
      }
      frame True {
      }
    }
    n321 = case shown="True" w173 {
      tunnel: w174 -> [_ w480]
      tunnel: [0.0 w480] -> w138
      frame False {
      }
      frame True {
      }
    }
    n322 = case shown="True" w149 {
      tunnel: w150 -> [_ w472]
      tunnel: [0.0 w472] -> w136
      frame False {
      }
      frame True {
      }
    }
    n323 = case shown="True" w257 {
      tunnel: w256 -> [_ w504]
      tunnel: [0.0 w504] -> w220
      frame False {
      }
      frame True {
      }
    }
    n324 = case shown="True" w235 {
      tunnel: w234 -> [_ w496]
      tunnel: [0.0 w496] -> w218
      frame False {
      }
      frame True {
      }
    }
    n325 = case shown="True" w249 {
      tunnel: w250 -> [_ w500]
      tunnel: [0.0 w500] -> w219
      frame False {
      }
      frame True {
      }
    }
    n326 = case shown="True" w274 {
      tunnel: w275 -> [_ w508]
      tunnel: [0.0 w508] -> w221
      frame False {
      }
      frame True {
      }
    }
    n327 = case shown="True" w314 {
      tunnel: w313 -> [_ w520]
      tunnel: [0.0 w520] -> w305
      frame False {
      }
      frame True {
      }
    }
    n328 = case shown="True" w283 {
      tunnel: w282 -> [_ w512]
      tunnel: [0.0 w512] -> w222
      frame False {
      }
      frame True {
      }
    }
    n329 = case shown="True" w326 {
      tunnel: w325 -> [_ w524]
      tunnel: [0.0 w524] -> w306
      frame False {
      }
      frame True {
      }
    }
    n330 = case shown="True" w201 {
      tunnel: w200 -> [_ w488]
      tunnel: [0.0 w488] -> w180
      frame False {
      }
      frame True {
      }
    }
    n331 = case shown="True" w298 {
      tunnel: w299 -> [_ w516]
      tunnel: [0.0 w516] -> w223
      frame False {
      }
      frame True {
      }
    }
    n332 = case shown="True" w338 {
      tunnel: w337 -> [_ w528]
      tunnel: [0.0 w528] -> w307
      frame False {
      }
      frame True {
      }
    }
    n333 = case shown="True" w352 {
      tunnel: w351 -> [_ w532]
      tunnel: [0.0 w532] -> w344
      frame False {
      }
      frame True {
      }
    }
    n334 = case shown="True" w212 {
      tunnel: w211 -> [_ w492]
      tunnel: [0.0 w492] -> w181
      frame False {
      }
      frame True {
      }
    }
    n335 = case shown="True" w365 {
      tunnel: w364 -> [_ w536]
      tunnel: [0.0 w536] -> w345
      frame False {
      }
      frame True {
      }
    }
    n336 = case shown="True" w188 {
      tunnel: w187 -> [_ w484]
      tunnel: [0.0 w484] -> w179
      frame False {
      }
      frame True {
      }
    }
    n337 = case shown="False" w378 {
      tunnel: w377 -> [_ w540]
      tunnel: [0.0 w540] -> w371
      frame False {
      }
      frame True {
      }
    }
    n338 = Build Array(w371, w345, w344, w307, w306, w305) -> (w372:dbl[])
    "7 Hz" <- w372
    n339 = Build Array(w454, w437, w424, w392, w385, w384) -> (w452:dbl[])
    "6 Hz" <- w452
    n340 = Array Max & Min(array=w372) -> (max value=w135:dbl, max index (indices)=→"Max Index 7":i32)  [unwired: 2 out]
    "PSD max 7" <- w135
    n341 = Array Max & Min(array=w452) -> (max value=w132:dbl, max index (indices)=→"Max Index 6":i32)  [unwired: 2 out]
    "PSD max 6" <- w132
    n342 = Build Array(w223, w222, w221, w220, w219, w218) -> (w224:dbl[])
    "8 Hz" <- w224
    n343 = Build Array(w181, w180, w179, w138, w137, w136) -> (w182:dbl[])
    "9 Hz" <- w182
    n344 = Array Max & Min(array=w224) -> (max value=w134:dbl, max index (indices)=→"Max Index 8":i32)  [unwired: 2 out]
    "PSD max 8" <- w134
    n345 = Array Max & Min(array=w182) -> (max value=w133:dbl, max index (indices)=→"Max Index 9":i32)  [unwired: 2 out]
    "PSD max 9" <- w133
    n346 = Build Array(w132, w135, w134, w133) -> (w131:dbl[])
    n347 = Array Max & Min(array=w131) -> (max value=w129:dbl, max index (indices)=w130:i32)  [unwired: 2 out]
    "max value" <- w129
    "PSD MAX" <- w129
    n348 = Greater?(x=w129, y=0.0 ("x")) -> (0:w127:bool)
    n349 = case shown="False" w127 {
      tunnel: w130 -> [_ w470]
      tunnel: [555 w470] -> w116
      frame False {
      }
      frame True {
      }
    }
    "Index ที่มากที่สุด" <- w116
    n350 = Equal?(x=0, y=w116) -> (x = y?=→"6 HZ":bool)
    n351 = Equal?(x=1, y=w116) -> (x = y?=→"7 HZ":bool)
    n352 = Equal?(x=2, y=w116) -> (x = y?=→"9 HZ":bool)
    n353 = Equal?(x=3, y=w116) -> (x = y?=→"8 HZ":bool)
    n354 = Equal?(x=555, y=w116) -> (x = y?=→"555":bool)
  }
  n355 = UDP Close(connection ID=w1, 8:w2) -> ()  [unwired: 2 out]
  n356 = while {
    stop <- FALSE stop-if-true
    n357 = event shown="[5] \"MENU 4\": Value Change" {
      selector: _ -> [_ _ _ _ _ _ _]
      dyn-events: _ -> [_ _ _ _ _ _ _]
      timeout: _ -> [_ _ _ _ _ _ _]
      event Timeout {
        n358 = event-data() -> ()  [unwired: 1 in, 3 out]
      }
      event "MENU": Value Change {
        n359 = event-data() -> ()  [unwired: 1 in, 6 out]
        n360 = local write "Tab Control"(enum32{"TAB 1", "TAB 2", "TAB 3", "TAB 4"}."TAB 2" ("Tab Control")) -> ()
      }
      event Value Change {
        n361 = event-data() -> ()  [unwired: 1 in, 6 out]
        n362 = local write "Tab Control"(enum32{"TAB 1", "TAB 2", "TAB 3", "TAB 4"}."TAB 1" ("Tab Control")) -> ()
      }
      event "MENU 2": Value Change {
        n363 = event-data() -> ()  [unwired: 1 in, 6 out]
        n364 = local write "Tab Control"(enum32{"TAB 1", "TAB 2", "TAB 3", "TAB 4"}."TAB 3" ("Tab Control")) -> ()
      }
      event "MENU 3": Value Change {
        n365 = event-data() -> ()  [unwired: 1 in, 6 out]
        n366 = local write "Tab Control"(enum32{"TAB 1", "TAB 2", "TAB 3", "TAB 4"}."TAB 4" ("Tab Control")) -> ()
      }
      event "MENU 4": Value Change {
        n367 = event-data() -> ()  [unwired: 1 in, 6 out]
        n368 = local write "Tab Control"(enum32{"TAB 1", "TAB 2", "TAB 3", "TAB 4"}."TAB 4" ("Tab Control")) -> ()
      }
      event "Back 4": Value Change {
        n369 = event-data() -> ()  [unwired: 1 in, 6 out]
        n370 = local write "Tab Control"(enum32{"TAB 1", "TAB 2", "TAB 3", "TAB 4"}."TAB 1" ("Tab Control")) -> ()
      }
    }
  }
  n371 = while {
    shift-right: [w583] -> _
    shift-left: "" -> [w585]
    stop <- FALSE stop-if-true
    n372 = event shown="[0] \"Text1\": Value Change" {
      selector: _ -> [_ _ _]
      dyn-events: _ -> [_ _ _]
      timeout: _ -> [_ _ _]
      tunnel: w585 -> [_ _ _]
      tunnel: ["ช่วยด้วย ฉันต้องการความช่วยเหลือ !!!" "ฉันต้องการรับประทานอาหาร" "ฉันมีโรคประจำตัว และรู้สึกอาการกำเริบ !!!"] -> w583
      event "Text1": Value Change {
        n373 = event-data() -> ()  [unwired: 1 in, 6 out]
      }
      event "Text2": Value Change {
        n374 = event-data() -> ()  [unwired: 1 in, 6 out]
      }
      event "Text3": Value Change {
        n375 = event-data() -> ()  [unwired: 1 in, 6 out]
      }
    }
    "String" <- w583
  }
  n376 = call-poly "VISA Configure Serial Port"("VISA resource name"="VISA resource name", "baud rate (9600)"=u32 9600) -> ("VISA resource name out"=w14:refnum<visa-resource-name>, "error out"=w12:errorcluster)  [unwired: 12 in]
  n377 = while {
    shift-right: [w597] -> w13
    shift-left: w14 -> [w598]
    shift-right: [w595] -> w11
    shift-left: w12 -> [w596]
    stop <- FALSE stop-if-true
    n378 = Select(t="a", s="LED", f="b") -> (s? t:f=w592:string)
    n379 = VISA Write(VISA resource name=w598, write buffer=w592, error in (no error)=w596) -> (VISA resource name out=w597:refnum<visa-resource-name>, error out=w595:errorcluster)  [unwired: 1 out]
    n380 = Wait (ms)(milliseconds to wait=u32 5) -> ()  [unwired: 1 out]
  }
  n381 = VISA Close(VISA resource name=w13, error in (no error)=w11) -> ()  [unwired: 1 out]
